vi "Deadzone.vi"(8 "error in":errorcluster, 10 "Input":dbl, 11 "Deadzone":dbl=0.05) -> (0 "error out":errorcluster, 2 "Output":dbl, 3 "In deadzone?":bool)   [LabVIEW 2015]
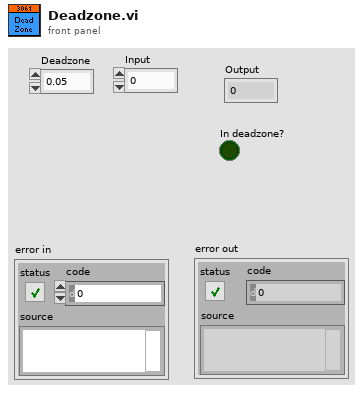
[diagram p1: front panel]
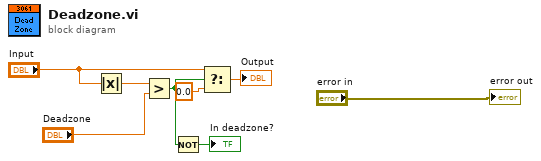
[diagram p0: block diagram]
diagram:
  n1 = Absolute Value(x="Input") -> (abs(x)=w8:dbl)
  n2 = Greater?(x=w8, y="Deadzone") -> (0:w7:bool)
  n3 = Not(x=w7) -> (.not. x?=→"In deadzone?":bool)
  n4 = Select(t="Input", s=w7, f=0.0) -> (s? t:f=→"Output":dbl)
  "error out" <- "error in"
